vi "Close.vi"(8 "error in (no error)":errorcluster, 11 "Motor-DAQmx in":refnum<class "Motor-DAQmx.lvclass">) -> (0 "error out":errorcluster, 3 "Motor-DAQmx out":refnum<class "Motor-DAQmx.lvclass">)   [LabVIEW 2013, in "PowderDeposition.lvlib" / "Motor-DAQmx.lvclass"]
uses:
  Motor-DAQmx.lvclass
  Motor-DAQmx.lvclass/Motor-DAQmx.ctl
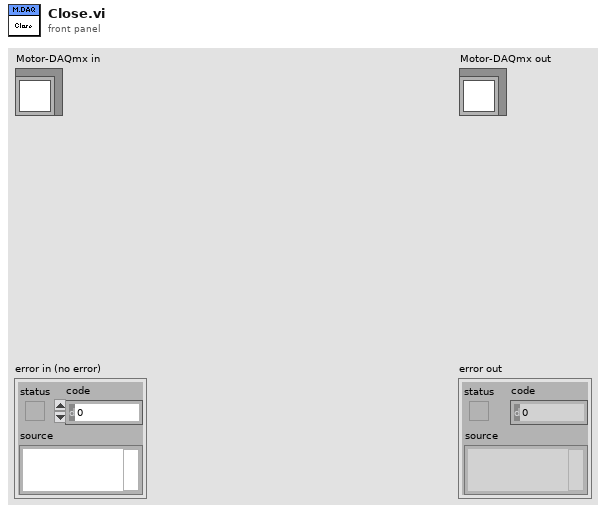
[diagram p1: front panel]
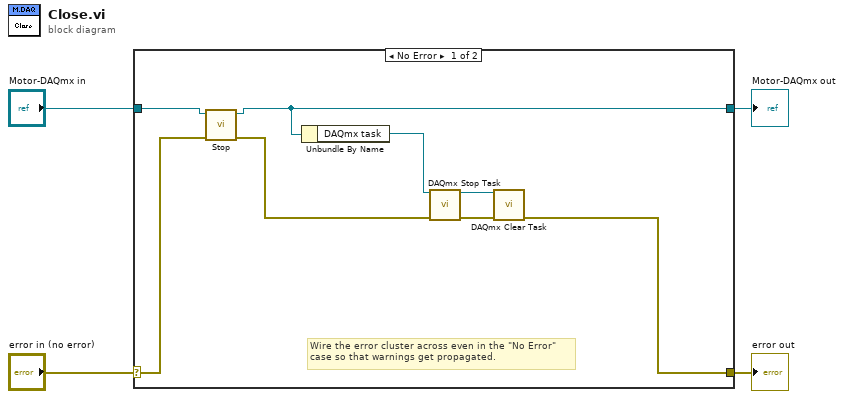
[diagram p0: block diagram]
diagram:
  n1 = case shown="No Error" "error in (no error)" {
    selector: "error in (no error)" -> [w8 w14]
    tunnel: [w5 w14] -> w3
    tunnel: [w11 w13] -> w1
    tunnel: "Motor-DAQmx in" -> [w12 w13]
    frame No Error {
      # "Wire the error cluster across even in the \"No Error\"\ncase so that warnings get propagated."
      n2 = call-dynamic "Stop.vi"("error in (no error)"=w8, "Motor-DAQmx in"=w12) -> ("error out"=w9:errorcluster, "Motor-DAQmx out"=w11:refnum<class "Motor-DAQmx.lvclass">)  [unwired: 8 in]
      n3 = Unbundle By Name(w11) -> ("DAQmx task"=w10:refnum<k21>)
      n4 = call <vilib>:"DAQmx Stop Task.vi"("task/channels in"=w10, "error in"=w9) -> ("task out"=w6:refnum<k21>, "error out"=w7:errorcluster)  [unwired: 12 in]
      n5 = call <vilib>:"DAQmx Clear Task.vi"("task in"=w6, "error in"=w7) -> ("error out"=w5:errorcluster)  [unwired: 13 in]
    }
    frame Error {
    }
  }
  "error out" <- w3
  "Motor-DAQmx out" <- w1
